vi "Load New Measurement.vi"(8 "error in (no error)":errorcluster, 11 "UI in":refnum<class "Measurement UI.lvclass">) -> (0 "error out":errorcluster, 3 "UI out":refnum<class "Measurement UI.lvclass">)   [LabVIEW 2015, in "Measurement UI.lvlib" / "Measurement UI.lvclass"]
uses:
  Msmt UI/Measurement UI.lvclass
  <vilib>/ActorFramework/Actor/Actor.lvclass/Actor.ctl
  Controller/Messages/Load Measurements/Find Measurements On Disk Message.lvclass
  Controller/Messages/Populate Mesaurements in UI/Display Measurements Message.lvclass
  <vilib>/ActorFramework/Actor/Actor.lvclass
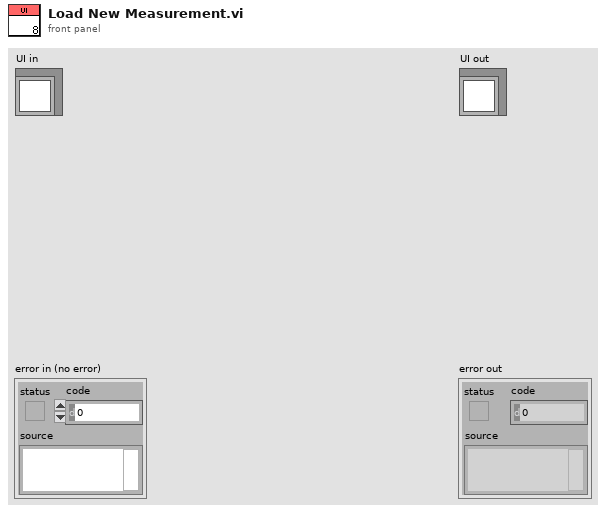
[diagram p1: front panel]
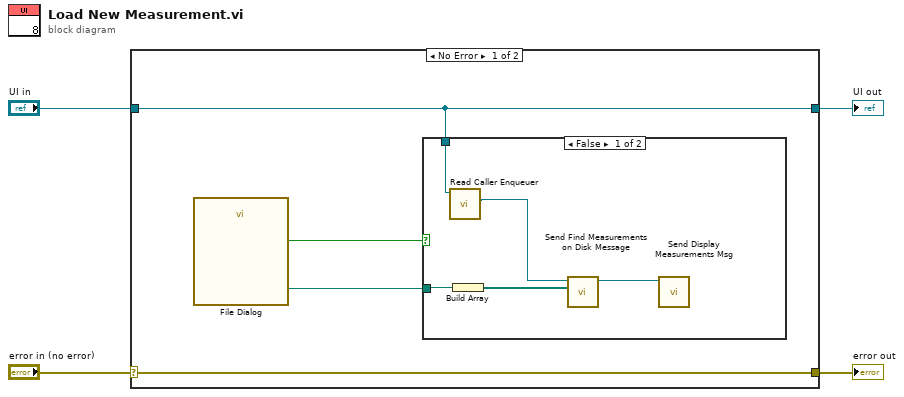
[diagram p0: block diagram]
diagram:
  n1 = case shown="No Error" "error in (no error)" {
    selector: "error in (no error)" -> [w8 w15]
    tunnel: [w8 w15] -> w3
    tunnel: [w5 w14] -> w1
    tunnel: "UI in" -> [w5 w14]
    frame No Error {
      n2 = call "File Dialog"() -> ("selected path"=w7:path, "cancelled"=w6:bool)  [unwired: 12 in, 2 out]
      n3 = case shown="False" w6 {
        tunnel: w7 -> [w10 _]
        tunnel: w5 -> [w12 _]
        frame False {
          n4 = call <vilib>:"Read Caller Enqueuer.vi"("Actor"=w12) -> ("Caller Enqueuer"=w11:refnum<class "Message Enqueuer.lvclass">)  [unwired: 10 in]
          n5 = Build Array(w10) -> (w9:path[])
          n6 = call "Send Find Measurements on Disk Message.vi"("Measurement Locations"=w9, "Message Enqueuer in"=w11) -> ("Message Enqueuer out"=w13:refnum<class "Message Enqueuer.lvclass">)  [unwired: 8 in, 1 out]
          n7 = call "Send Display Measurements Msg.vi"("Message Enqueuer in"=w13) -> ()  [unwired: 9 in, 2 out]
        }
        frame True {
        }
      }
    }
    frame Error {
    }
  }
  "error out" <- w3
  "UI out" <- w1
